vi "Sign In Example.vi"() -> ()   [LabVIEW 2019]
uses:
  firebase.lvclass
panel:
  out "firebase out":refnum<class "firebase.lvclass">
  in  "Email":string
  in  "Password":string
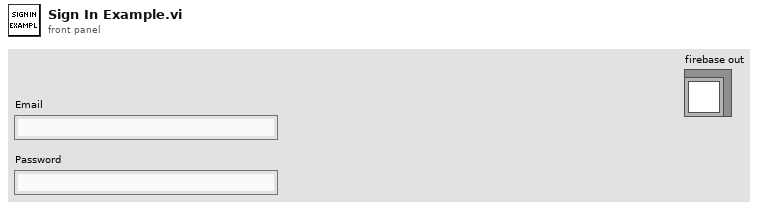
[diagram p1: front panel]
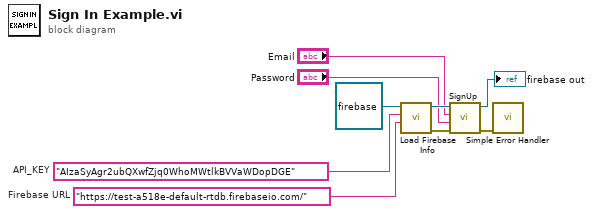
[diagram p0: block diagram]
diagram:
  w1 = "AIzaSyAgr2ubQXwfZjq0WhoMWtlkBVVaWDopDGE"  # API_KEY
  w2 = "https://test-a518e-default-rtdb.firebaseio.com/"  # Firebase URL
  n1 = call "Load Firebase Info.vi"("Firebase URL"=w2, "API_KEY"=w1, "firebase in"=refnum<class "firebase.lvclass"> refnum ("firebase.lvclass")) -> ("error out"=w9:errorcluster, "firebase out"=w6:refnum<class "firebase.lvclass">)  [unwired: 7 in]
  n2 = call-dynamic "SignUp.vi"("error in"=w9, "password"="Password", "email"="Email", "firebase in"=w6) -> ("error out"=w8:errorcluster, "firebase out"=→"firebase out":refnum<class "firebase.lvclass">)  [unwired: 6 in]
  n3 = call <vilib>:"Simple Error Handler.vi"("error in (no error)"=w8) -> ()  [unwired: 4 in, 5 out]
